vi "Sender.vi"() -> ()   [LabVIEW 2021]
panel:
  out "Bytes Written":dbl
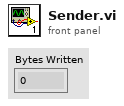
[diagram p1: front panel]
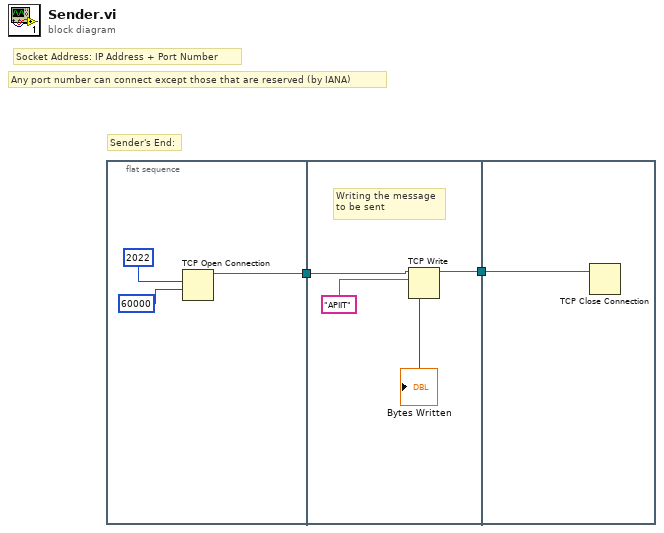
[diagram p0: block diagram]
diagram:
  # "Sender's End:"
  # "Any port number can connect except those that are reserved (by IANA)"
  # "Socket Address: IP Address + Port Number"
  n1 = flat-sequence {
    tunnel: [w3] -> w2
    tunnel: w2 -> [w9]
    tunnel: [w6] -> w1
    tunnel: w1 -> [w10]
    frame #0 {
      n2 = TCP Open Connection(remote port or service name=2022, timeout ms (60000)=60000) -> (connection ID=w3:refnum<k5>)  [unwired: 3 in, 1 out]
    }
    frame #1 {
      # "Writing the message\nto be sent"
      n3 = TCP Write(connection ID=w9, data in="APIIT") -> (connection ID out=w6:refnum<k5>, bytes written=→"Bytes Written":i32)  [unwired: 2 in, 1 out]
    }
    frame #2 {
      n4 = TCP Close Connection(connection ID=w10) -> ()  [unwired: 2 in, 2 out]
    }
  }
